vi "Init SubPanel Dialog.vi"(7 "SubPanel in":refnum<class "SubPanel.lvclass">, 8 "error in (no error)":errorcluster, 10 "VI Path":path, 11 "MsgBox Title":string) -> (0 "error out":errorcluster, 3 "SubPanel out":refnum<class "SubPanel.lvclass">)   [LabVIEW 2012, in "SubPanel.lvlib" / "SubPanel.lvclass"]
uses:
  SubPanel.lvclass
  MessageBox/pictures/pictures.ctl
  SubPanel.lvclass/SubPanel.ctl
  MessageBox/MessageBox.lvclass
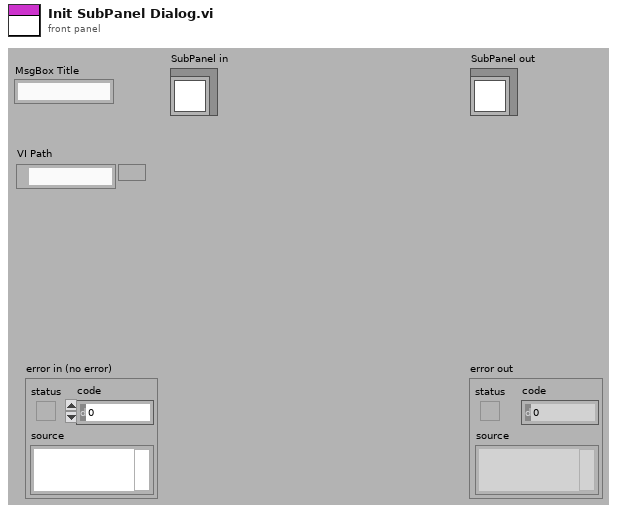
[diagram p1: front panel]
types:
  T1 = typedef "pictures.ctl" = enum16{"Alarm", "Download", "Edition", "Encrypted", "Error", "Hardware Information", "Important", "Memory", "Network", "Package", "Password", "Readme", "Search", "System", "USB", "User", "Wireless", "www"}
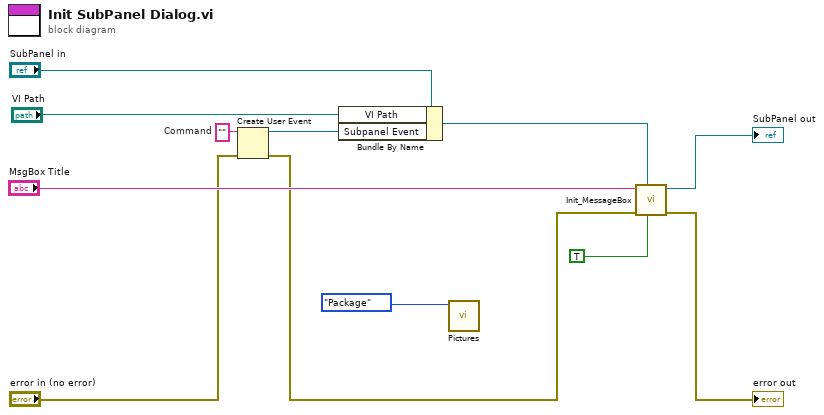
[diagram p0: block diagram]
diagram:
  w4 = ""  # Command
  n1 = Create User Event(user event datatype=w4, error in="error in (no error)") -> (user event=w3:refnum<user-event>, error out=w1:errorcluster)
  n2 = Bundle By Name(cluster="SubPanel in", "VI Path"="VI Path", "Subpanel Event"=w3) -> (w7:refnum<class "SubPanel.lvclass">)
  n3 = call "Pictures.vi"("Pictures"=pictures."Package") -> ()  [unwired: 11 out]
  n4 = call "Init_MessageBox.vi"("Allow to close? (T)"=TRUE, "MessageBox in"=w7, "error in (no error)"=w1, "MsgBox Title"="MsgBox Title") -> ("error out"=→"error out":errorcluster, "MessageBox out"=→"SubPanel out":refnum<class "SubPanel.lvclass">)  [unwired: 3 in, 3 out]
